vi "LocalScriptFilename.vi"() -> (0 "Filename Out":path)   [LabVIEW 2014]
doc: "Use this template to build a standard state machine design pattern. Each state executes code and determines which state to transition to. Contrast this design pattern with the user interface event pattern, in which code executes in response to user actions. Contrast this design pattern also with the queued message handler pattern, in which each message handling code can queue zero or more new messages."
panel:
  in  "Filename":path
  in  "Close":bool
  in  "Run":bool
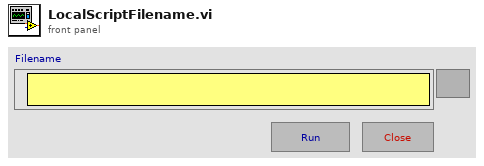
[diagram p1: front panel]
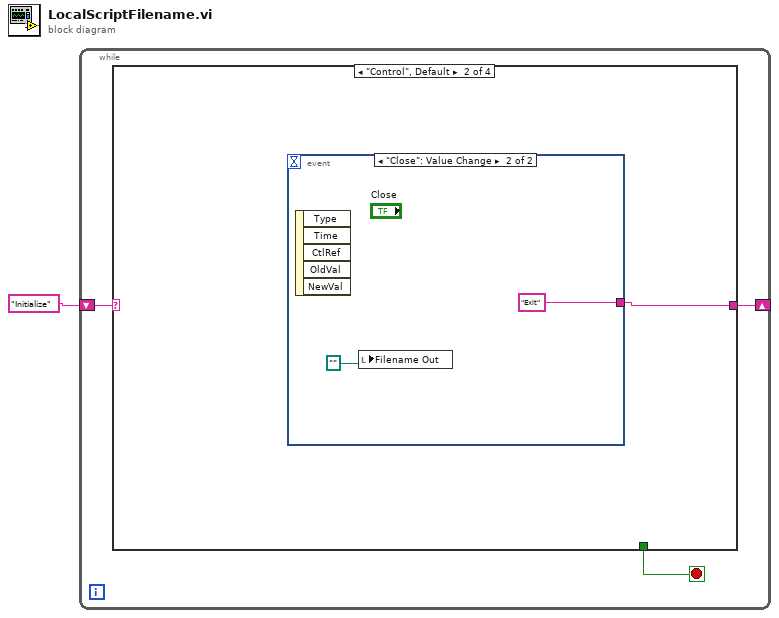
[diagram p0: block diagram]
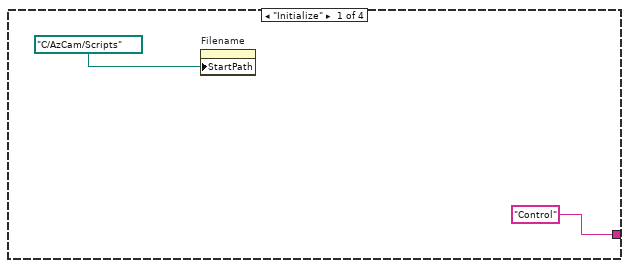
[diagram p2: hidden frame]
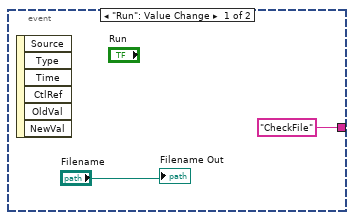
[diagram p3: hidden frame]
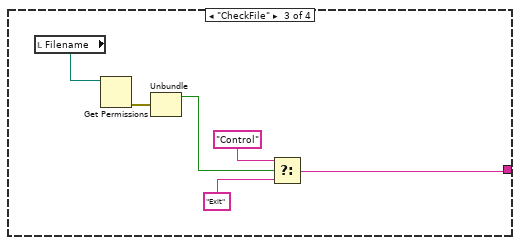
[diagram p4: hidden frame]
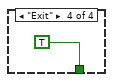
[diagram p5: hidden frame]
diagram:
  n1 = while {
    shift-right: [w2] -> _
    shift-left: "Initialize" -> [w3]
    stop <- w4 stop-if-true
    n2 = case shown="\"Control\", Default" w3 {
      tunnel: [_ _ _ TRUE] -> w4
      tunnel: ["Control" w7 w12 _] -> w2
      frame "Initialize" {
        n3 = property on="Filename" class="Path"("StartPath"=path "C:/AzCam/Scripts" ("Browse Options:Start Path")) -> ()  [unwired: 2 in, 2 out]
      }
      frame "Control", Default {
        n4 = event shown="[1] \"Close\": Value Change" {
          selector: _ -> [_ _]
          dyn-events: _ -> [_ _]
          timeout: _ -> [_ _]
          tunnel: ["CheckFile" "Exit"] -> w7
          event "Run": Value Change {
            n5 = event-data() -> ()  [unwired: 1 in, 6 out]
            "Filename Out" <- "Filename"
          }
          event "Close": Value Change {
            n6 = event-data() -> ()  [unwired: 1 in, 5 out]
            n7 = local write "Filename Out"(path "") -> ()
          }
        }
      }
      frame "CheckFile" {
        n8 = local read "Filename"() -> (w17:path)
        n9 = Get Permissions(11:w17) -> (0:w16:errorcluster)  [unwired: 1 in, 4 out]
        n10 = Unbundle(w16) -> ("status"=w15:bool)  [unwired: 2 out]
        n11 = Select(t="Control", s=w15, f="Exit") -> (s? t:f=w12:string)
      }
      frame "Exit" {
      }
    }
  }
